vi "Set Symbol.vi"(7 "Skip If Worse (F)":bool, 8 "error in (no error)":errorcluster, 9 "Test Outcome":T1, 10 "Tag Name":string, 11 "ResultTree in":refnum<class "Result Tree.lvclass">) -> (0 "error out":errorcluster, 3 "ResultTree out":refnum<class "Result Tree.lvclass">)   [LabVIEW 2017, in "Result Tree.lvclass"]
doc: "Sets the symbol for the specified tag name based on the provided test outcome. The default behavior is to skip tags whose outcome is already worse than the provided outcome."
uses:
  Result Tree.lvclass
  Test Outcome.ctl
  Result Tree.lvclass/Result Tree.ctl
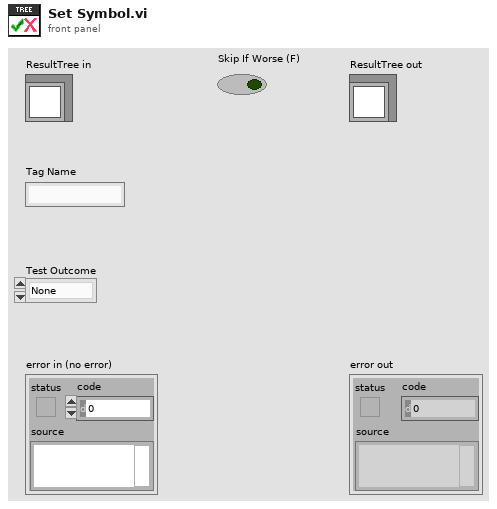
[diagram p1: front panel]
types:
  T1 = typedef "Test Outcome.ctl" = enum16{"None", "Passed", "Failed"}
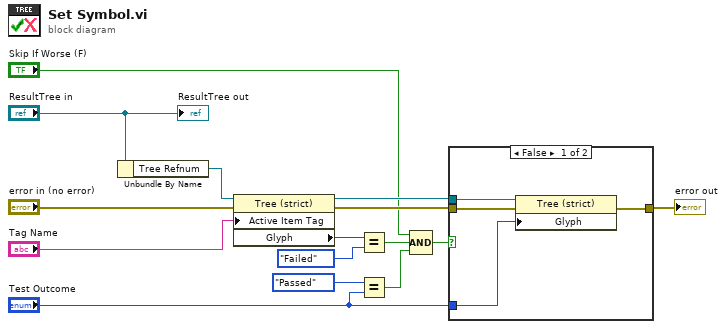
[diagram p0: block diagram]
diagram:
  n1 = Unbundle By Name("ResultTree in") -> ("Tree Refnum"=w13:refnum<vi>)
  n2 = property class="Tree (strict)"(reference=w13, error in="error in (no error)", "Active Item Tag"="Tag Name") -> (reference out=w9:refnum<vi>, error out=w11:errorcluster, "Glyph"=w6:i32)
  n3 = Equal?(x=w6, y=Test_Outcome."Failed" ("Test Outcome")) -> (x = y?=w2:bool)
  n4 = Equal?(x=Test_Outcome."Passed", y="Test Outcome") -> (x = y?=w1:bool)
  n5 = Compound Arithmetic op=AND("Skip If Worse (F)", w2, w1) -> (w8:bool)
  n6 = case shown="False" w8 {
    tunnel: [w19 w20] -> w15
    tunnel: "Test Outcome" -> [w18 _]
    tunnel: w11 -> [w17 w20]
    tunnel: w9 -> [w16 _]
    frame False {
      n7 = property class="Tree (strict)"(reference=w16, error in=w17, "Glyph"=w18) -> (error out=w19:errorcluster)  [unwired: 1 out]
    }
    frame True {
    }
  }
  "error out" <- w15
  "ResultTree out" <- "ResultTree in"
